vi "serverNewTcpListenerID.vi"(8 "error in (no error)":errorcluster, 11 "tcpServer in":refnum<class "TcpServer.lvclass">) -> (0 "error out":errorcluster, 3 "tcpServer out":refnum<class "TcpServer.lvclass">)   [LabVIEW 2018, in "TcpServer.lvclass"]
doc: "Create a new tcp Listener ID."
uses:
  TcpServer.lvclass
  TcpServer.lvclass/TcpServer.ctl
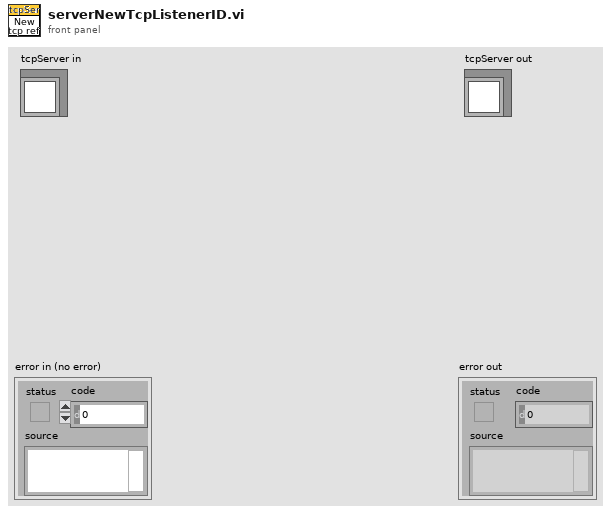
[diagram p1: front panel]
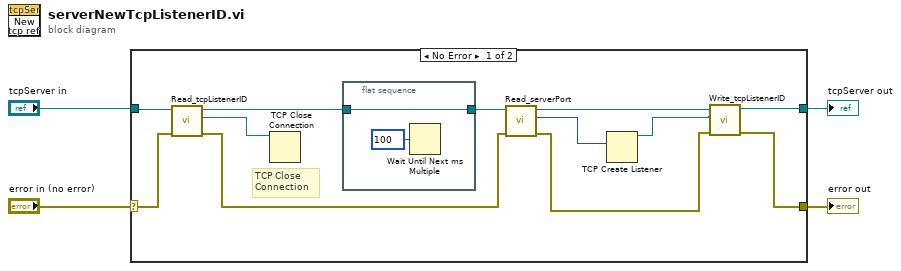
[diagram p0: block diagram]
diagram:
  n1 = case shown="No Error" "error in (no error)" {
    selector: "error in (no error)" -> [w14 w20]
    tunnel: [w5 w20] -> w3
    tunnel: [w16 w19] -> w1
    tunnel: "tcpServer in" -> [w15 w19]
    frame No Error {
      # "TCP Close \nConnection"
      n2 = call "Read_tcpListenerID.vi"("error in (no error)"=w14, "tcpServer in"=w15) -> ("error out"=w7:errorcluster, "tcpListenerID"=w13:refnum<k5>, "tcpServer out"=w9:refnum<class "TcpServer.lvclass">)  [unwired: 7 in]
      n3 = TCP Close Connection(connection ID=w13) -> ()  [unwired: 2 in, 2 out]
      n4 = flat-sequence {
        tunnel: w9 -> [w17]
        tunnel: [w17] -> w8
        frame #0 {
          n5 = Wait Until Next ms Multiple(millisecond multiple=100) -> ()  [unwired: 1 out]
        }
      }
      n6 = call "Read_serverPort.vi"("error in (no error)"=w7, "tcpServer in"=w8) -> ("error out"=w6:errorcluster, "serverPort"=w12:u16, "tcpServer out"=w11:refnum<class "TcpServer.lvclass">)  [unwired: 7 in]
      n7 = TCP Create Listener(10:w12) -> (3:w10:refnum<k5>)  [unwired: 4 in, 2 out]
      n8 = call "Write_tcpListenerID.vi"("error in (no error)"=w6, "tcpListenerID"=w10, "tcpServer in"=w11) -> ("error out"=w5:errorcluster, "tcpServer out"=w16:refnum<class "TcpServer.lvclass">)  [unwired: 7 in]
    }
    frame Error {
    }
  }
  "error out" <- w3
  "tcpServer out" <- w1
